vi "Peak_Max_Update_subVI.vi"(11 "Measurement Cluster":T1) -> (3 "Measurement Cluster Out":T1)   [LabVIEW 2015]
uses:
  --Controls and TypeDefs--/Measurement_Cluster.ctl
  --Controls and TypeDefs--/Raman_Model_Data_Cluster.ctl
panel:
  # "Flow Rate Measurements"
  # "Temp Measurements"
  # "Raman Measurements"
  # "Flow Rate Measurements"
  # "Temp Measurements"
  # "Raman Measurements"
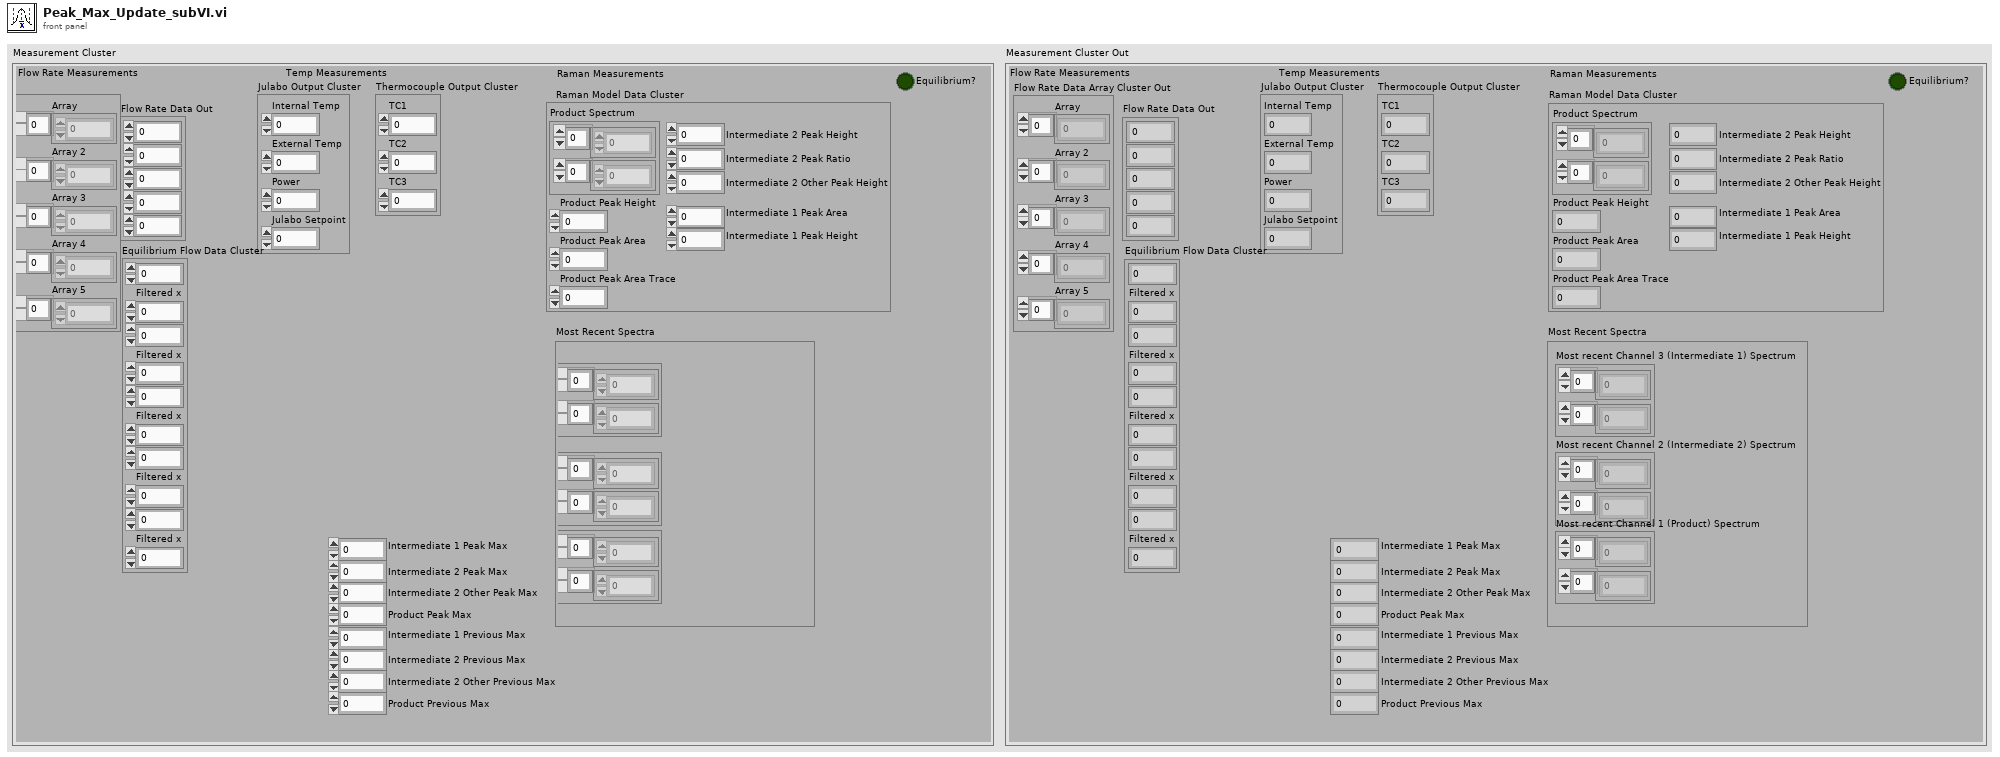
[diagram p1: front panel]
types:
  T1 = typedef "Measurement_Cluster.ctl" = cluster{"Raman Model Data Cluster":T2, "Julabo Output Cluster":cluster{"Internal Temp":dbl, "External Temp":dbl, "Power":i8, "Julabo Setpoint":dbl}, "Thermocouple Output Cluster":cluster{"TC1":dbl, "TC2":dbl, "TC3":dbl}, "Flow Rate Data Array Cluster Out":cluster{"Array":dbl[], "Array 2":dbl[], "Array 3":dbl[], "Array 4":dbl[], "Array 5":dbl[]}, "Flow Rate Data Out":cluster{dbl, dbl, dbl, dbl, dbl}, "Equilibrium?":bool, "Equilibrium Flow Data Cluster":cluster{dbl, "Filtered x":dbl, dbl, "Filtered x":dbl, dbl, "Filtered x":dbl, dbl, "Filtered x":dbl, dbl, "Filtered x":dbl}, "Most Recent Spectra":cluster{"Most recent Channel 3 (Intermediate 1) Spectrum":cluster{i32[], i32[]}, "Most recent Channel 2 (Intermediate 2) Spectrum":cluster{i32[], i32[]}, "Most recent Channel 1 (Product) Spectrum":cluster{i32[], i32[]}}, "Intermediate 2 Other Peak Max":i32, "Intermediate 2 Peak Max":i32, "Intermediate 1 Peak Max":i32, "Product Peak Max":i32, "Intermediate 2 Other Previous Max":i32, "Intermediate 2 Previous Max":i32, "Intermediate 1 Previous Max":i32, "Product Previous Max":i32}
  T2 = typedef "Raman_Model_Data_Cluster.ctl" = cluster{"Product Spectrum":cluster{i32[], i32[]}, "Product Peak Height":i32, "Product Peak Area":i32, "Product Peak Area Trace":i32, "Intermediate 2 Peak Height":i32, "Intermediate 1 Peak Area":i32, "Intermediate 1 Peak Height":i32, "Intermediate 2 Other Peak Height":i32, "Intermediate 2 Peak Ratio":i32}
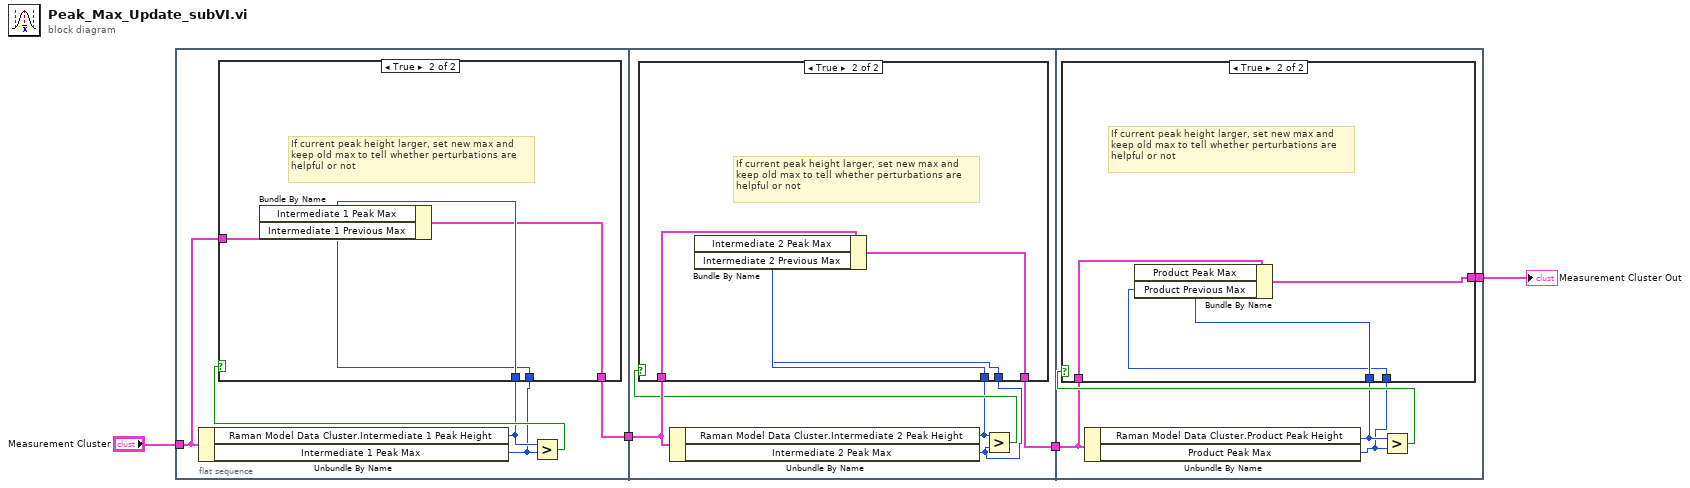
[diagram p0: block diagram]
diagram:
  n1 = flat-sequence {
    tunnel: "Measurement Cluster" -> [w8]
    tunnel: [w6] -> w3
    tunnel: w3 -> [w19]
    tunnel: [w17] -> w2
    tunnel: w2 -> [w28]
    tunnel: [w27] -> w1
    frame #0 {
      n2 = Unbundle By Name(w8) -> ("Raman Model Data Cluster.Intermediate 1 Peak Height"=w7:i32, "Intermediate 1 Peak Max"=w5:i32)
      n3 = Greater?(x=w7, y=w5) -> (0:w9:bool)
      n4 = case shown="True" w9 {
        tunnel: w8 -> [w10 w14]
        tunnel: w7 -> [_ w13]
        tunnel: [w10 w12] -> w6
        tunnel: w5 -> [_ w11]
        frame False {
        }
        frame True {
          # "If current peak height larger, set new max and\nkeep old max to tell whether perturbations are\nhelpful or not"
          n5 = Bundle By Name(cluster=w14, "Intermediate 1 Peak Max"=w13, "Intermediate 1 Previous Max"=w11) -> (w12:T1)
        }
      }
    }
    frame #1 {
      n6 = Unbundle By Name(w19) -> ("Raman Model Data Cluster.Intermediate 2 Peak Height"=w16:i32, "Intermediate 2 Peak Max"=w15:i32)
      n7 = Greater?(x=w16, y=w15) -> (0:w18:bool)
      n8 = case shown="True" w18 {
        tunnel: w19 -> [w20 w24]
        tunnel: [w20 w22] -> w17
        tunnel: w16 -> [_ w23]
        tunnel: w15 -> [_ w21]
        frame False {
        }
        frame True {
          # "If current peak height larger, set new max and\nkeep old max to tell whether perturbations are\nhelpful or not"
          n9 = Bundle By Name(cluster=w24, "Intermediate 2 Peak Max"=w23, "Intermediate 2 Previous Max"=w21) -> (w22:T1)
        }
      }
    }
    frame #2 {
      n10 = Unbundle By Name(w28) -> ("Raman Model Data Cluster.Product Peak Height"=w26:i32, "Product Peak Max"=w25:i32)
      n11 = Greater?(x=w26, y=w25) -> (0:w29:bool)
      n12 = case shown="True" w29 {
        tunnel: w28 -> [w30 w34]
        tunnel: [w30 w32] -> w27
        tunnel: w26 -> [_ w33]
        tunnel: w25 -> [_ w31]
        frame False {
        }
        frame True {
          # "If current peak height larger, set new max and\nkeep old max to tell whether perturbations are\nhelpful or not"
          n13 = Bundle By Name(cluster=w34, "Product Peak Max"=w33, "Product Previous Max"=w31) -> (w32:T1)
        }
      }
    }
  }
  "Measurement Cluster Out" <- w1
